vi "Generate sweep.vi"(5 "input dt":dbl, 7 "samples":i32, 11 "Current treatment":T1) -> (1 "vel":dbl[](array[numeric]), 2 "pos":dbl[](array[numeric]), 3 "Treatment out":T1)   [LabVIEW 2012]
uses:
  Treatment.ctl
  Treatment type.ctl
  <vilib>/Analysis/3filter.llb/Filter Passband Type.ctl
  <vilib>/Analysis/1siggen.llb/Ramp Pattern by Samples.vi
  <vilib>/Analysis/NI_AALBase.lvlib
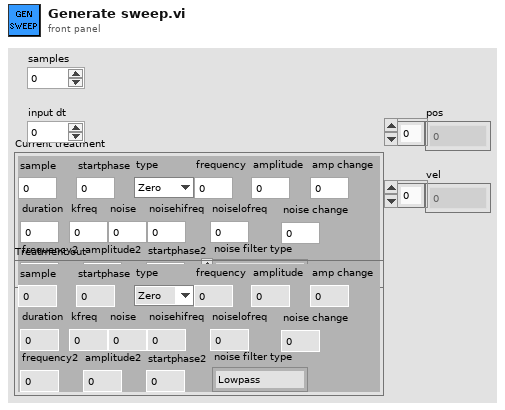
[diagram p1: front panel]
types:
  T1 = typedef "Treatment.ctl" = cluster{"sample":dbl, "startphase":dbl, "type":T2, "frequency":dbl, "amplitude":dbl, "noise":dbl, "duration":dbl, "kfreq":dbl, "noisehifreq":dbl, "frequency2":dbl, "amplitude2":dbl, "startphase2":dbl, "noise filter type":T3, "noiselofreq":dbl, "amp change":dbl, "noise change":dbl}
  T2 = typedef "Treatment type.ctl" = enum16{"Zero", "Sine", "Frequency sweep", "Two frequency", "Amplitude sweep"}
  T3 = typedef "NI_AALBase.lvlib/Filter Passband Type.ctl" = enum32{"Lowpass", "Highpass", "Bandpass", "Bandstop"}
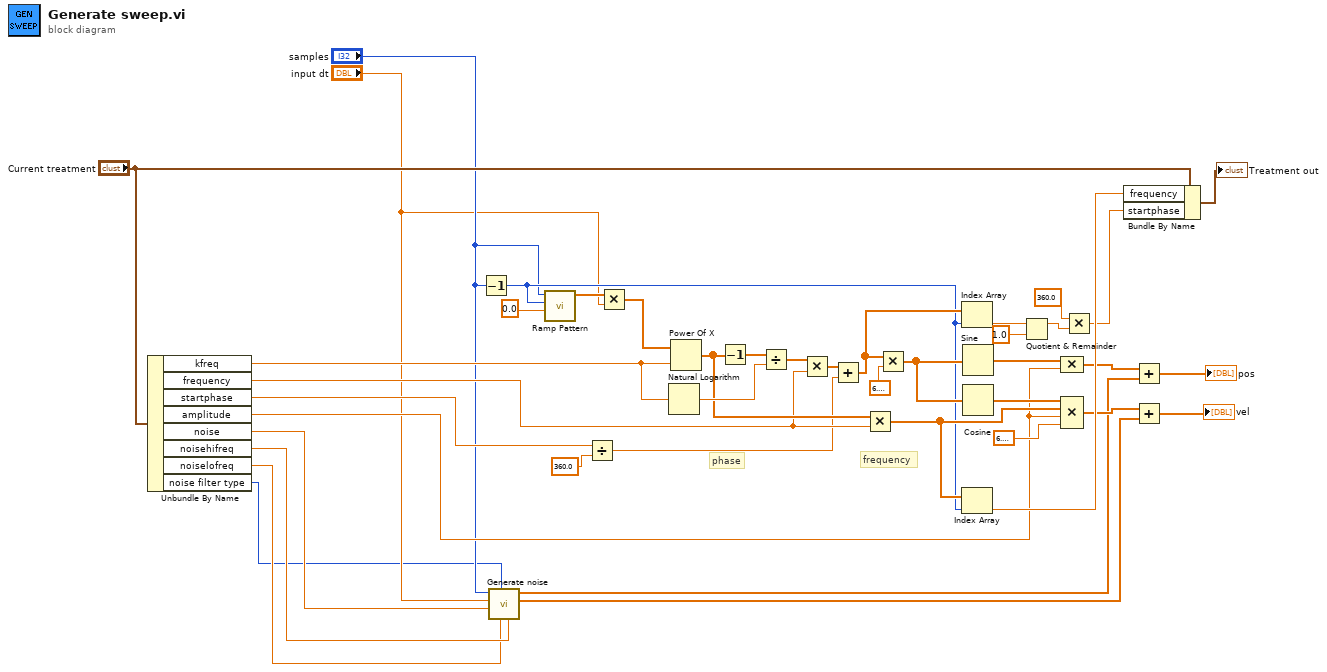
[diagram p0: block diagram]
diagram:
  # "frequency"
  # "phase"
  n1 = Unbundle By Name("Current treatment") -> ("kfreq"=w39:dbl, "frequency"=w34:dbl, "startphase"=w22:dbl, "amplitude"=w16:dbl, "noise"=w13:dbl, "noisehifreq"=w3:dbl, "noiselofreq"=w2:dbl, "noise filter type"=w1:T3)
  n2 = Decrement(x="samples") -> (x-1=w20:i32)
  n3 = call "Generate noise.vi"("noisehifreq"=w3, "noiselofreq"=w2, "filter type"=w1, "noise std"=w13, "input dt"="input dt", "samples"="samples") -> ("noise deriv"=w11:dbl[], "noise"=w12:dbl[])  [unwired: 4 in]
  n4 = call-poly <vilib>:"Ramp Pattern.vi"("start"=0.0, "end"=w20, "samples"="samples") -> ("Ramp Pattern"=w24:dbl[])  [unwired: 7 in, 1 out]
  n5 = Divide(x=w22, y=360.0) -> (x/y=w5:dbl)
  n6 = Multiply(x=w24, y="input dt") -> (x*y=w25:dbl[])
  n7 = Natural Logarithm(1:w39) -> (0:w37:dbl)
  n8 = Power Of X(1:w39, 2:w25) -> (0:w35:dbl[])
  n9 = Decrement(x=w35) -> (x-1=w38:dbl[])
  n10 = Divide(x=w38, y=w37) -> (x/y=w36:dbl[])
  n11 = Multiply(x=w36, y=w34) -> (x*y=w23:dbl[])
  n12 = Add(x=w23, y=w5) -> (x+y=w21:dbl[])
  n13 = Multiply(x=w35, y=w34) -> (x*y=w30:dbl[])
  n14 = Multiply(x=w21, y=6.283185307179586) -> (x*y=w32:dbl[])
  n15 = Index Array(array=w21, index=w20) -> (element=w10:dbl)
  n16 = Index Array(array=w30, index=w20) -> (element=w29:dbl)
  n17 = Sine(x=w32) -> (sin(x)=w19:dbl[])
  n18 = Cosine(x=w32) -> (cos(x)=w31:dbl[])
  n19 = Quotient & Remainder(x=w10, y=1.0) -> (x-y*floor(x/y)=w9:dbl)  [unwired: 1 out]
  n20 = Compound Arithmetic op=MULTIPLY(w19, w16) -> (w18:dbl[])
  n21 = Compound Arithmetic op=MULTIPLY(w31, w30, w16, 6.283185307179586) -> (w28:dbl[])
  n22 = Multiply(x=360.0, y=w9) -> (x*y=w7:dbl)
  n23 = Bundle By Name(cluster="Current treatment", "frequency"=w29, "startphase"=w7) -> (→"Treatment out":T1)
  n24 = Add(x=w18, y=w12) -> (x+y=→"pos":dbl[])
  n25 = Add(x=w28, y=w11) -> (x+y=→"vel":dbl[])
